vi "Post Installer Actions.vi"   [LabVIEW 2014]
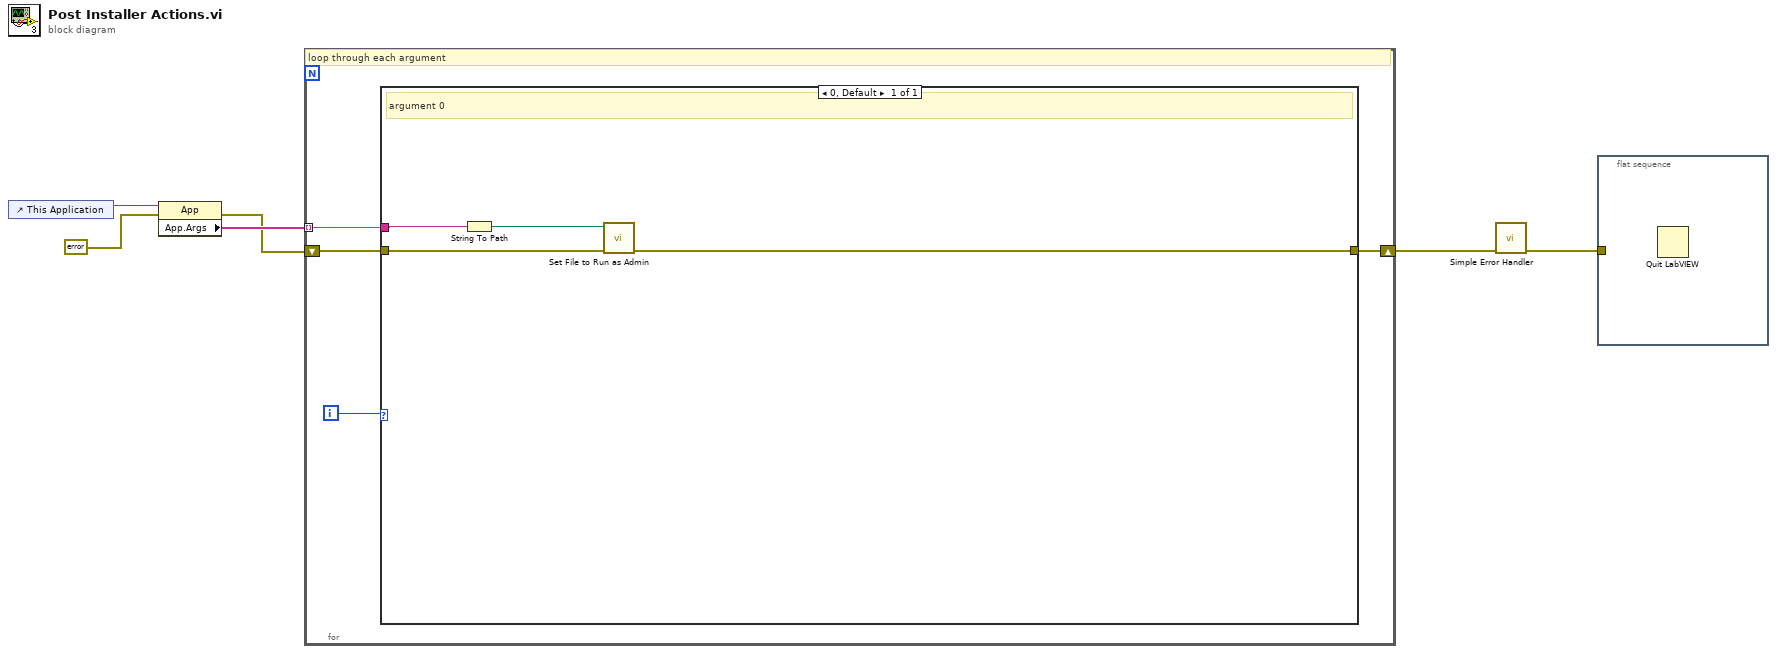
[diagram p0: block diagram]
diagram:
  n1 = control-ref of="This Application"() -> (w6:refnum<vi>)
  n2 = property class="App"(reference=w6, error in=errorcluster {"status"=FALSE, "code"=0, "source"=""} ("error in (no error)")) -> (error out=w3:errorcluster, "App.Args"=w4:string[])  [unwired: 1 out]
  n3 = for {
    tunnel: w4 -> [w9] mode=indexing
    shift-right: [w7] -> w2
    shift-left: w3 -> [w8]
    i -> [w10]
    # "loop through each argument"
    n4 = case shown="0, Default" w10 {
      tunnel: w9 -> [w14]
      tunnel: w8 -> [w12]
      tunnel: [w11] -> w7
      frame 0, Default {
        # "argument 0"
        n5 = String To Path(string=w14) -> (path=w13:path)
        n6 = call "Set File to Run as Admin.vi"("Error In"=w12, "Path to file that needs to be run as admin"=w13) -> ("Error Out"=w11:errorcluster)  [unwired: 9 in]
      }
    }
  }
  n7 = call <vilib>:"Simple Error Handler.vi"("error in (no error)"=w2) -> ("error out"=w1:errorcluster)  [unwired: 4 in, 4 out]
  n8 = flat-sequence {
    tunnel: w1 -> [_]
    frame #0 {
      n9 = Quit LabVIEW() -> ()  [unwired: 1 in]
    }
  }
